vi "LEDSetpoint.vi"() -> ()   [LabVIEW 2018]
uses:
  Actions.ctl
panel:
  in  "Action":T1
  in  "Height Setpoint":dbl
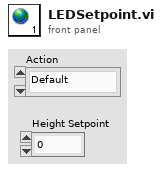
[diagram p1: front panel]
types:
  T1 = typedef "Actions.ctl" = enum16{"Default", "Hatch Triggered", "Lost Vision", "Auto Aiming", "Party Mode", "Has Hatch", "Brownout", "Height Setpoint"}
diagram:
